vi "Set Tenney SM1.vi"(0 "Interface\nType":refnum<visa-resource-name>="Tenney35", 2 "Temp,Humidity ChartOut":refnum<vi>, 5 "Temp Set Point":dbl, 7 "Humidity Set Point":dbl, 11 "Error In":errorcluster) -> (4 "Chamber Stable":bool, 6 "Set Point Reached":bool, 15 "Error Out":errorcluster)   [LabVIEW 2009]
panel:
  out "H Reset":bool
  out "Temp reset":bool
  in  "Stability Time(s)":i32=14400
  out "Temp,Humidity Chart":T1(graph)
  out "Actual Humidity Readback (%)":dbl format="%.2f"
  out "Actual Temp Readback (C)":dbl format="%.2f"
  in  "Time Limit(seconds)":i32=14400
  out "Temp Reached":bool
  out "Humid. reached":bool
  in  "Humid. Band":dbl
  in  "Temp Band":dbl
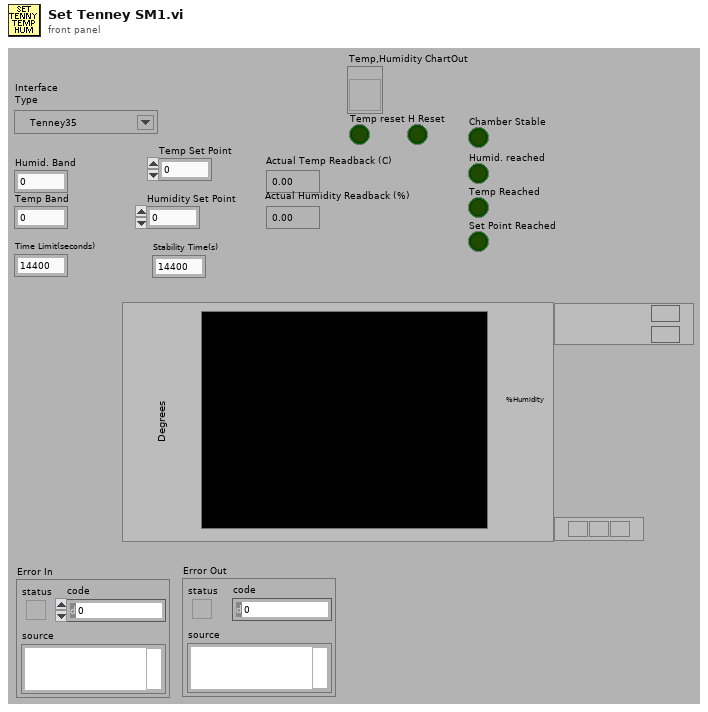
[diagram p1: front panel]
types:
  T1 = cluster{"[0]":dbl, "[1]":dbl, "[2]":dbl, "[3]":dbl, "[4]":dbl, "[5]":dbl}
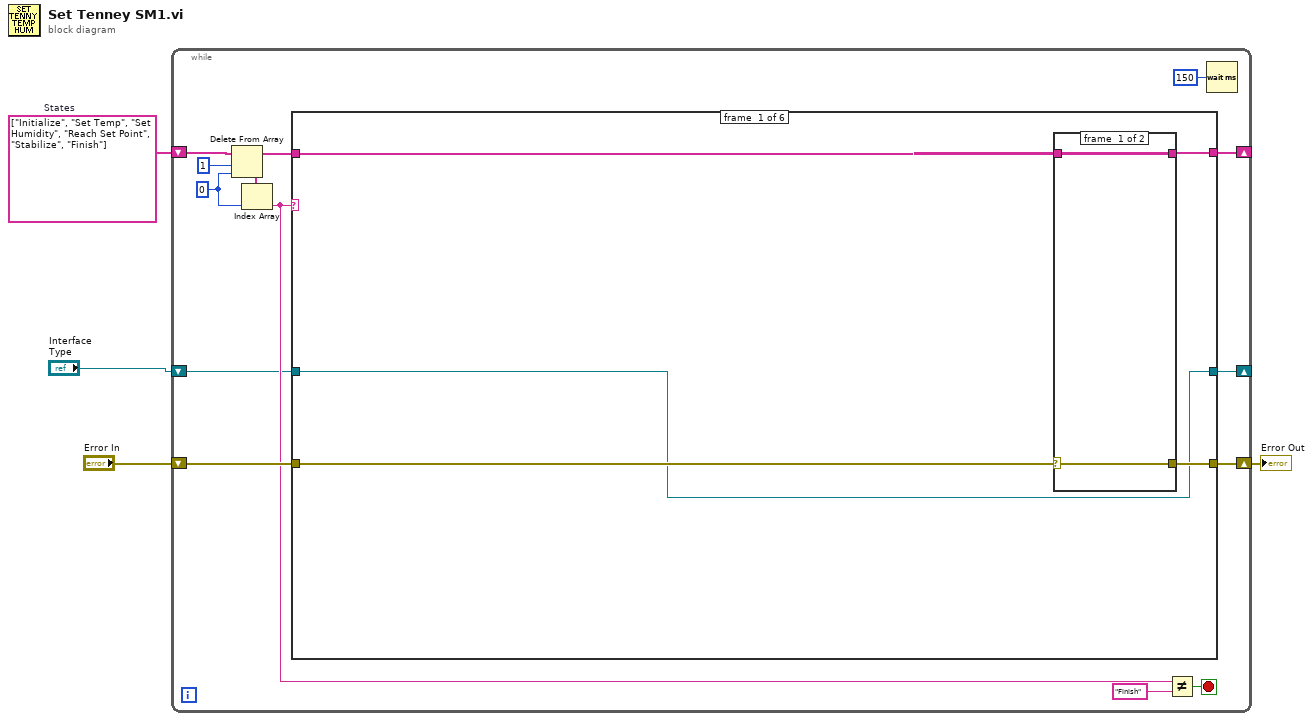
[diagram p0: block diagram]
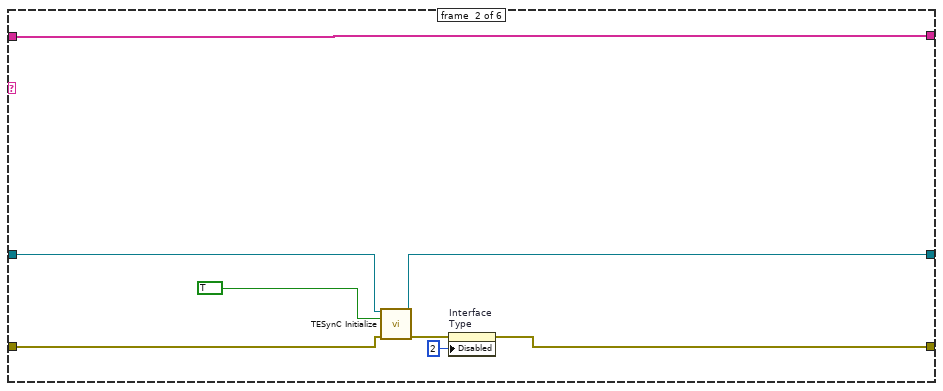
[diagram p3: hidden frame]
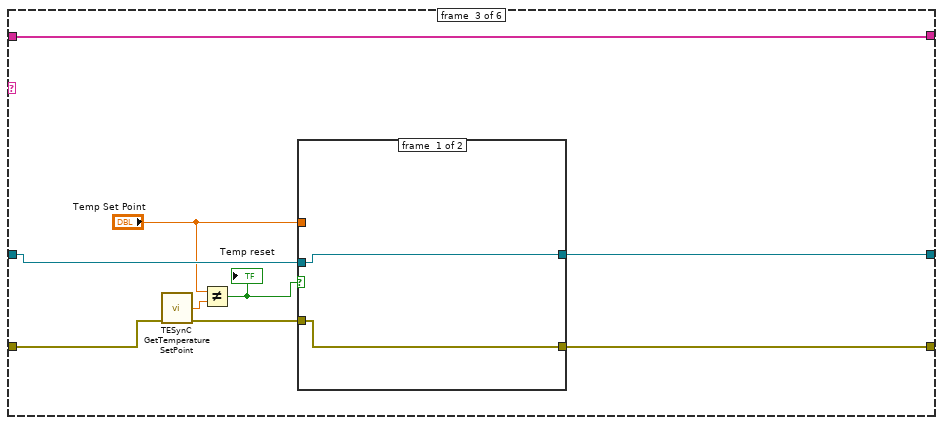
[diagram p4: hidden frame]
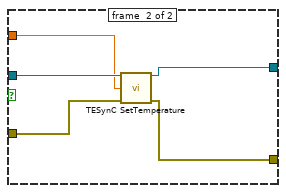
[diagram p5: hidden frame]
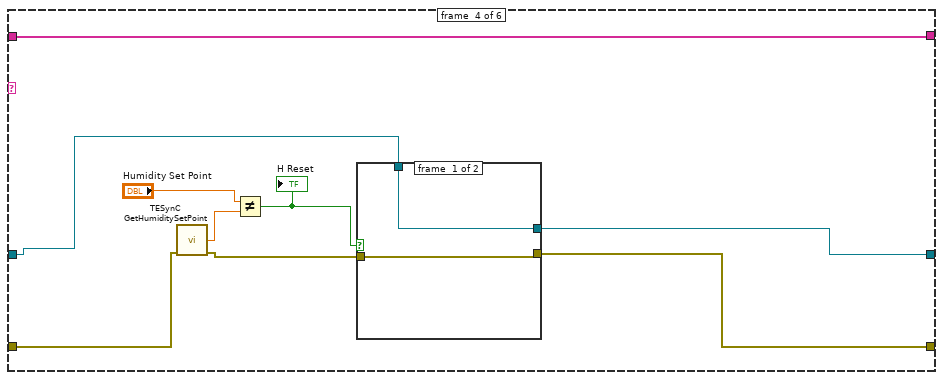
[diagram p6: hidden frame]
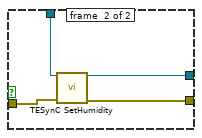
[diagram p7: hidden frame]
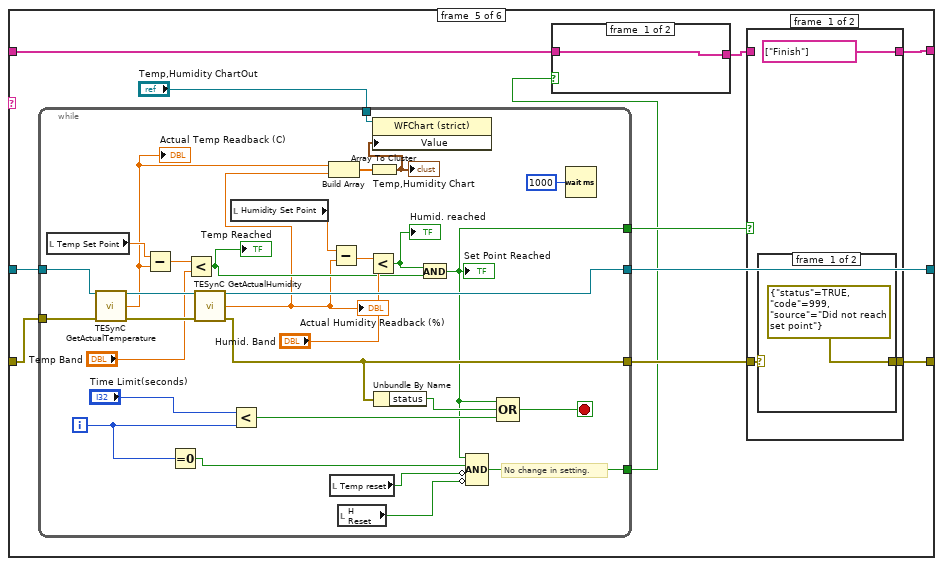
[diagram p8: hidden frame]
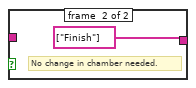
[diagram p9: hidden frame]
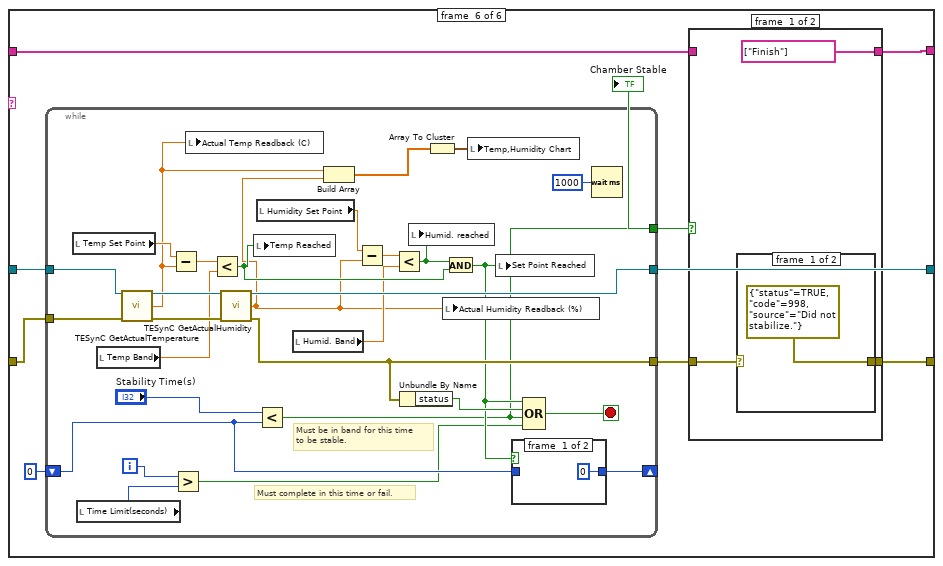
[diagram p12: hidden frame]
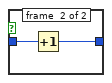
[diagram p15: hidden frame]
diagram:
  w4 = string[] ["Initialize", "Set Temp", "Set Humidity", "Reach Set Point", "Stabilize", "Finish"]  # States
  n1 = while {
    shift-right: [w14] -> _
    shift-left: w4 -> [w18]
    shift-right: [w11] -> w2
    shift-left: "Error In" -> [w10]
    shift-right: [w6] -> _
    shift-left: "Interface\nType" -> [w5]
    stop <- w9 stop-if-true
    w15 = 0 ("index")
    n2 = Delete From Array(array=w18, length=1, index=w15) -> (deleted portion=w16:string[], array with subset deleted=w13:string[])
    n3 = Index Array(array=w16, index=w15) -> (element=w8:string)
    n4 = case shown="\"Reach Set Point\"" w8 {
      tunnel: [w23 w35 w36 w53 w74 w122] -> w14
      tunnel: w13 -> [w22 w35 w36 w53 w68 w121]
      tunnel: [w21 w30 w42 w56 w73 w120] -> w11
      tunnel: w10 -> [w20 w31 w41 w58 w77 w125]
      tunnel: [w19 w29 w44 w55 w75 w123] -> w6
      tunnel: w5 -> [w19 w28 w43 w54 w76 w124]
      frame #0 {
        n5 = case shown="Error" w20 {
          selector: w20 -> [w24 w26]
          tunnel: [w25 w27] -> w23
          tunnel: w22 -> [w25 w27]
          tunnel: [w24 w26] -> w21
          frame #0 {
          }
          frame #1 {
          }
        }
      }
      frame #1 {
        n6 = call "TESynC Initialize.vi"("VISA resource name"=w28, "ID Query (T: Check)"=TRUE, "error in (no error)"=w31) -> ("VISA session"=w29:refnum<visa-resource-name>, "error out"=w34:errorcluster)  [unwired: 11 in]
        n7 = property on="Interface\nType" class="VISAName"(error in=w34, "Disabled"=u8 2) -> (error out=w30:errorcluster)  [unwired: 1 in, 1 out]
      }
      frame #2 {
        n8 = call "TESynC GetTemperatureSetPoint.vi"("error in (no error)"=w41) -> ("Temp Setpoint Readback (C)"=w40:dbl, "error out"=w38:errorcluster)  [unwired: 12 in, 1 out]
        n9 = Not Equal?(x="Temp Set Point", y=w40) -> (x != y?=w39:bool)
        "Temp reset" <- w39
        n10 = case shown="True" w39 {
          tunnel: [w45 w51] -> w44
          tunnel: w43 -> [w45 w50]
          tunnel: [w46 w49] -> w42
          tunnel: w38 -> [w46 w48]
          tunnel: "Temp Set Point" -> [_ w47]
          frame #0 {
          }
          frame #1 {
            n11 = call "TESynC SetTemperature.vi"("VISA session in"=w50, "Temperature (C"=w47, "error in (no error)"=w48) -> ("VISA session out"=w51:refnum<visa-resource-name>, "error out"=w49:errorcluster)  [unwired: 11 in]
          }
        }
      }
      frame #3 {
        n12 = call "TESynC GetHumiditySetPoint.vi"("error in (no error)"=w58) -> ("Setpoint Humidity Readback(%)"=w60:dbl, "error out"=w57:errorcluster)  [unwired: 12 in, 1 out]
        n13 = Not Equal?(x="Humidity Set Point", y=w60) -> (x != y?=w59:bool)
        "H Reset" <- w59
        n14 = case shown="False" w59 {
          tunnel: w57 -> [w61 w66]
          tunnel: [w61 w65] -> w56
          tunnel: [w62 w64] -> w55
          tunnel: w54 -> [w62 w63]
          frame #0 {
          }
          frame #1 {
            n15 = call "TESynC SetHumidity.vi"("VISA session in"=w63, "error in (no error)"=w66) -> ("VISA session out"=w64:refnum<visa-resource-name>, "error out"=w65:errorcluster)  [unwired: 12 in]
          }
        }
      }
      frame #4 {
        n16 = while {
          tunnel: w77 -> [w116]
          tunnel: w76 -> [w112]
          tunnel: [w110] -> w75
          tunnel: [w102] -> w72
          tunnel: [w93] -> w71
          tunnel: [w89] -> w70
          tunnel: "Temp,Humidity ChartOut" -> [w88]
          i -> [w94]
          stop <- w98 stop-if-true
          # "No change in setting."
          n17 = local read "Temp Set Point"() -> (w113:dbl)
          n18 = call "TESynC GetActualTemperature.vi"("VISA session in"=w112, "error in (no error)"=w116) -> ("VISA session out"=w111:refnum<visa-resource-name>, "Actual Temp Readback (C)"=w96:dbl, "error out"=w115:errorcluster)  [unwired: 11 in]
          "Actual Temp Readback (C)" <- w96
          n19 = Subtract(x=w113, y=w96) -> (x-y=w109:dbl)
          n20 = Equal To 0?(x=w94) -> (x = 0?=w92:bool)
          n21 = Less?(x=w109, y="Temp Band") -> (x < y?=w104:bool)
          "Temp Reached" <- w104
          n22 = call "TESynC GetActualHumidity.vi"("VISA session in"=w111, "error in (no error)"=w115) -> ("VISA session out"=w110:refnum<visa-resource-name>, "Actual Humidity Readback (%)"=w97:dbl, "error out"=w102:errorcluster)  [unwired: 11 in]
          "Actual Humidity Readback (%)" <- w97
          n23 = local read "Humidity Set Point"() -> (w114:dbl)
          n24 = Less?(x="Time Limit(seconds)", y=w94) -> (x < y?=w99:bool)
          n25 = Build Array(w96, w97) -> (w95:dbl[])
          n26 = local read "Temp reset"() -> (w91:bool)
          n27 = Subtract(x=w114, y=w97) -> (x-y=w107:dbl)
          n28 = local read "H Reset"() -> (w90:bool)
          n29 = Less?(x=w107, y="Humid. Band") -> (x < y?=w105:bool)
          "Humid. reached" <- w105
          n30 = Array To Cluster(array=w95) -> (cluster=w87:T1)
          "Temp,Humidity Chart" <- w87
          n31 = property on="Property Node" class="WFChart (strict)"(reference=w88, "Value"=w87) -> ()  [unwired: 1 in, 2 out]
          n32 = Unbundle By Name(w102) -> ("status"=w101:bool)
          n33 = And(x=w105, y=w104) -> (x .and. y?=w93:bool)
          "Set Point Reached" <- w93
          n34 = Compound Arithmetic op=AND(w93, w92, invert w91, invert w90) -> (w89:bool)
          n35 = Compound Arithmetic op=OR(w93, w101, w99) -> (w98:bool)
          n36 = Wait (ms)(milliseconds to wait=u32 1000) -> ()  [unwired: 1 out]
        }
        n37 = case shown="False" w70 {
          tunnel: [w78 string[] ["Finish"] ("States")] -> w69
          tunnel: w68 -> [w78 _]
          frame #0 {
          }
          frame #1 {
            # "No change in chamber needed."
          }
        }
        n38 = case shown="True" w71 {
          tunnel: [string[] ["Finish"] ("States") w86] -> w74
          tunnel: w69 -> [_ w86]
          tunnel: [w81 w85] -> w73
          tunnel: w72 -> [w80 w85]
          frame #0 {
            n39 = case shown="No Error" w80 {
              selector: w80 -> [_ w84]
              tunnel: [errorcluster {"status"=TRUE, "code"=999, "source"="Did not reach set point"} ("error IO") w84] -> w81
              frame #0 {
              }
              frame #1 {
              }
            }
          }
          frame #1 {
          }
        }
      }
      frame #5 {
        n40 = while {
          tunnel: w125 -> [w161]
          tunnel: w124 -> [w157]
          tunnel: [w155] -> w123
          tunnel: [w152] -> w119
          tunnel: [w133] -> w118
          shift-right: [w136] -> _
          shift-left: 0 -> [w135]
          i -> [w139]
          stop <- w149 stop-if-true
          # "Must be in band for this time\nto be stable."
          # "Must complete in this time or fail."
          n41 = local read "Temp Set Point"() -> (w158:dbl)
          n42 = local read "Time Limit(seconds)"() -> (w138:i32)
          n43 = local read "Temp Band"() -> (w143:dbl)
          n44 = call "TESynC GetActualTemperature.vi"("VISA session in"=w157, "error in (no error)"=w161) -> ("VISA session out"=w156:refnum<visa-resource-name>, "Actual Temp Readback (C)"=w144:dbl, "error out"=w160:errorcluster)  [unwired: 11 in]
          n45 = Subtract(x=w158, y=w144) -> (x-y=w154:dbl)
          n46 = Greater?(x=w139, y=w138) -> (0:w134:bool)
          n47 = local write "Actual Temp Readback (C)"(w144) -> ()
          n48 = Less?(x=w154, y=w143) -> (x < y?=w145:bool)
          n49 = call "TESynC GetActualHumidity.vi"("VISA session in"=w156, "error in (no error)"=w160) -> ("VISA session out"=w155:refnum<visa-resource-name>, "Actual Humidity Readback (%)"=w140:dbl, "error out"=w152:errorcluster)  [unwired: 11 in]
          n50 = local write "Temp Reached"(w145) -> ()
          n51 = local read "Humidity Set Point"() -> (w159:dbl)
          n52 = Less?(x="Stability Time(s)", y=w135) -> (x < y?=w133:bool)
          n53 = local read "Humid. Band"() -> (w142:dbl)
          n54 = Build Array(w144, w140) -> (w148:dbl[])
          n55 = Subtract(x=w159, y=w140) -> (x-y=w141:dbl)
          n56 = Less?(x=w141, y=w142) -> (x < y?=w146:bool)
          n57 = Unbundle By Name(w152) -> ("status"=w151:bool)
          n58 = local write "Humid. reached"(w146) -> ()
          n59 = Array To Cluster(array=w148) -> (cluster=w147:T1)
          n60 = local write "Actual Humidity Readback (%)"(w140) -> ()
          n61 = And(x=w146, y=w145) -> (x .and. y?=w137:bool)
          n62 = local write "Temp,Humidity Chart"(w147) -> ()
          n63 = local write "Set Point Reached"(w137) -> ()
          n64 = case shown="False" w137 {
            tunnel: [0 w164] -> w136
            tunnel: w135 -> [_ w163]
            frame #0 {
            }
            frame #1 {
              n65 = Increment(x=w163) -> (x+1=w164:i32)
            }
          }
          n66 = Compound Arithmetic op=OR(w137, w151, w133, w134) -> (w149:bool)
          n67 = Wait (ms)(milliseconds to wait=u32 1000) -> ()  [unwired: 1 out]
        }
        "Chamber Stable" <- w118
        n68 = case shown="False" w118 {
          tunnel: [string[] ["Finish"] ("States") w132] -> w122
          tunnel: w121 -> [_ w132]
          tunnel: [w127 w131] -> w120
          tunnel: w119 -> [w126 w131]
          frame #0 {
            n69 = case shown="No Error" w126 {
              selector: w126 -> [_ w130]
              tunnel: [errorcluster {"status"=TRUE, "code"=998, "source"="Did not stabilize."} ("error IO") w130] -> w127
              frame #0 {
              }
              frame #1 {
              }
            }
          }
          frame #1 {
          }
        }
      }
    }
    n70 = Not Equal?(x=w8, y="Finish") -> (x != y?=w9:bool)
    n71 = Wait (ms)(milliseconds to wait=u32 150) -> ()  [unwired: 1 out]
  }
  "Error Out" <- w2
